vi "Create and Read Output Tags.vi"() -> ()   [LabVIEW 2020]
uses:
  <vilib>/Skyline/Tag/Shared/typedefs/DataType.ctl
  <vilib>/Skyline/Tag/Wrapper/Wrapper AMQP_class/Open Tag AMQP.vi
  <vilib>/Skyline/Tag/Wrapper/Wrapper_class/Read Tag (DBL).vi
  <vilib>/Skyline/Tag/Wrapper/Wrapper_class/Close Tag (Single).vi
  FlexLoggerTagHelpers.lvlib
  <vilib>/Skyline/Tag/Wrapper/Wrapper_class/NI Skyline Tag.lvclass
  <vilib>/Skyline/Tag/Shared/NI Skyline Tag.lvlib
  <vilib>/Skyline/Tag/Wrapper/Wrapper AMQP_class/NI Skyline Tag AMQP.lvclass
panel:
  out "Value":dbl
  in  "Channel Name":string="My Test Channel"
  in  "Group Name":string="My Test Group"
  in  "Stop":bool
  # "Overview: This example demonstrates using SystemLink tags as outputs which can be controlled from FlexLogger.\nRequirements: LabVIEW Full Development System, FlexLogger\nInstructions:\n1. Launch FlexLogger\n     a. Create a Project     \n     b. Using the Project >> Settings menu, enable Publish SystemLink Tags (Export) and Consume External SystemLink Tags (Import)\n     c. Restart the FlexLogger Project\n2. Run this VI.\n3. Add a screen control and map it to the channel corresponding to the name specified on the front panel below.\n4. Change the value of the screen control and observe updates to the value on the front panel below."
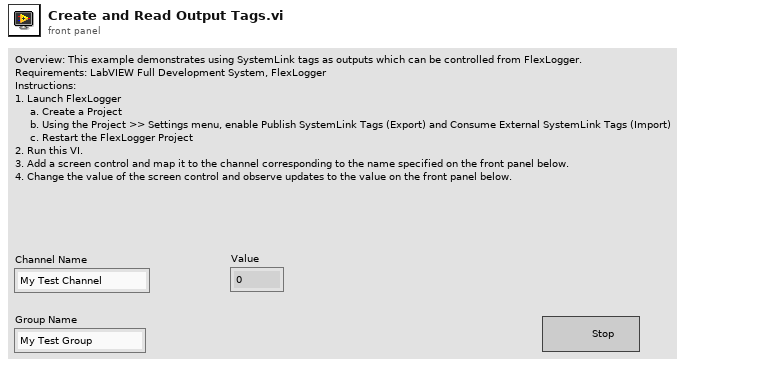
[diagram p1: front panel]
types:
  T1 = typedef "NI Skyline Tag.lvlib/DataType.ctl" = enum32{"Double", "I32", "String", "Boolean", "U64", "Timestamp"}
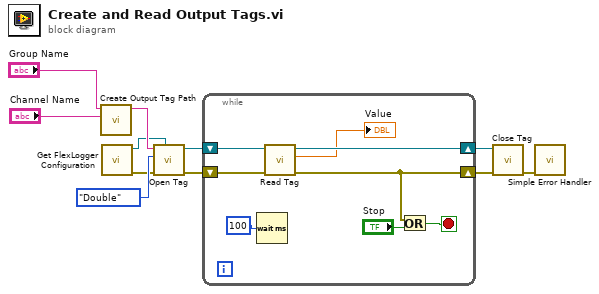
[diagram p0: block diagram]
diagram:
  n1 = call "Create Output Tag Path.vi"("Channel Name"="Channel Name", "Group Name"="Group Name") -> ("Path"=w11:string)  [unwired: 9 in]
  n2 = call "Get FlexLogger Configuration.vi"() -> ("error out"=w2:errorcluster, "Local FlexLogger Configuration"=w1:refnum<class "NI Skyline Configuration AMQP.lvclass">)  [unwired: 10 in]
  n3 = call-poly <vilib>:"Open Tag.vi"("configuration"=w1, "error in (no error)"=w2, "data type"=DataType."Double", "path"=w11) -> ("error out"=w6:errorcluster, "tag"=w9:refnum<class "NI Skyline Tag.lvclass">)  [unwired: 6 in]
  n4 = while {
    shift-right: [w14] -> w5
    shift-left: w9 -> [w17]
    shift-right: [w15] -> w4
    shift-left: w6 -> [w16]
    stop <- w18 stop-if-true
    n5 = Wait (ms)(milliseconds to wait=u32 100) -> ()  [unwired: 1 out]
    n6 = call-poly <vilib>:"Read Tag.vi"("error in (no error)"=w16, "tag in"=w17) -> ("error out"=w15:errorcluster, "value"=→"Value":dbl, "tag out"=w14:refnum<class "NI Skyline Tag.lvclass">)  [unwired: 5 in, 2 out]
    n7 = Or(x=w15, y="Stop") -> (x .or. y?=w18:bool)
  }
  n8 = call-poly <vilib>:"Close Tag.vi"("error in (no error)"=w4, "tag"=w5) -> ("error out"=w3:errorcluster)  [unwired: 9 in]
  n9 = call <vilib>:"Simple Error Handler.vi"("error in (no error)"=w3) -> ()  [unwired: 4 in, 5 out]
